vi "Download DSP402 (U8).vi"(4 "error in (no error)":errorcluster, 5 "Value":u8, 6 "Multiplexor":T1 {"Sub-Index" format="%.0x"; "Index" format="%04x"}, 7 "DSP402 in":refnum<class "DSP402.lvclass">) -> (0 "error out":errorcluster, 3 "DSP402 out":refnum<class "DSP402.lvclass">)   [LabVIEW 2026, in "canopen_.lvlib" / "DSP402.lvclass"]
uses:
  DSP402.lvclass
  DSP402.lvclass/DSP402.ctl
  CANopen/CANopen.lvclass
  CANopen/SDO download (U8).vi
  CANopen/Multiplexor.ctl
  CANopen Master.lvlib
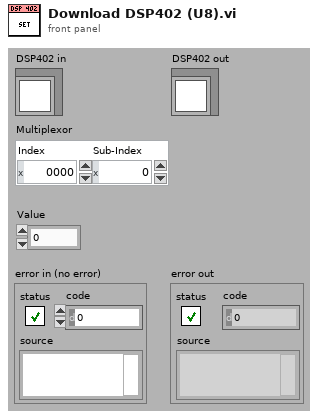
[diagram p1: front panel]
types:
  T1 = typedef "CANopen Master.lvlib/Multiplexor.ctl" = cluster{"Index":u16, "Sub-Index":i16}
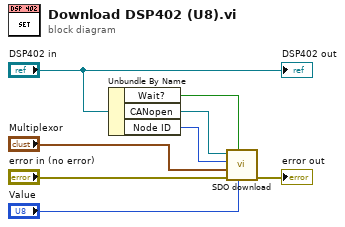
[diagram p0: block diagram]
diagram:
  n1 = Unbundle By Name("DSP402 in") -> ("Wait?"=w3:bool, "CANopen"=w6:refnum<class "CANopen.lvclass">, "Node ID"=w5:u8)
  n2 = call-poly "SDO download.vi"("Value"="Value", "Wait?"=w3, "error in (no error)"="error in (no error)", "Multiplexor"="Multiplexor", "Node ID"=w5, "CANopen in"=w6) -> ("error out"=→"error out":errorcluster)  [unwired: 3 out]
  "DSP402 out" <- "DSP402 in"
